vi "LCR_Logfile.vi"(4 "Data cluster":T1, 6 "Time Stamp":timestamp format="%<%x %.3X>T", 8 "error in":errorcluster, 9 "Data_In":T2 {"GUI Data Cluster"."SBR" format="%08b"}, 10 "Config_In":T4={"General"={"Config.ini"=path "", "Default Logging Path"=path ""}, "Hardware"={"Global T VAR"="", "Global B VAR"="", "VISAS"={"GEN COM"="", "SCOPE COM"="", "VNA COM"=""}}, "Operation"={"Operation Mode"=enum."Idle-Off", "Status"="", "NewLog?"=FALSE, "OvenWarn"=FALSE, "Scope Settings"={"TimeBase"=0.0, "VerticalScale"=4.0}}}) -> (0 "error out":errorcluster, 1 "Data_Out":T2 {"GUI Data Cluster"."SBR" format="%08b"}, 2 "Config_Out":T4={"General"={"Config.ini"=path "", "Default Logging Path"=path ""}, "Hardware"={"Global T VAR"="", "Global B VAR"="", "VISAS"={"GEN COM"="", "SCOPE COM"="", "VNA COM"=""}}, "Operation"={"Operation Mode"=enum."Idle-Off", "Status"="", "NewLog?"=FALSE, "OvenWarn"=FALSE, "Scope Settings"={"TimeBase"=0.0, "VerticalScale"=4.0}}}, 3 "File Failure":bool)   [LabVIEW 2021]
uses:
  Config_Cluster.ctl
  Mode_Enum.ctl
  Data_Cluster.ctl
  Measurement_Cluster.ctl
panel:
  in  "Status Ref":refnum<vi>
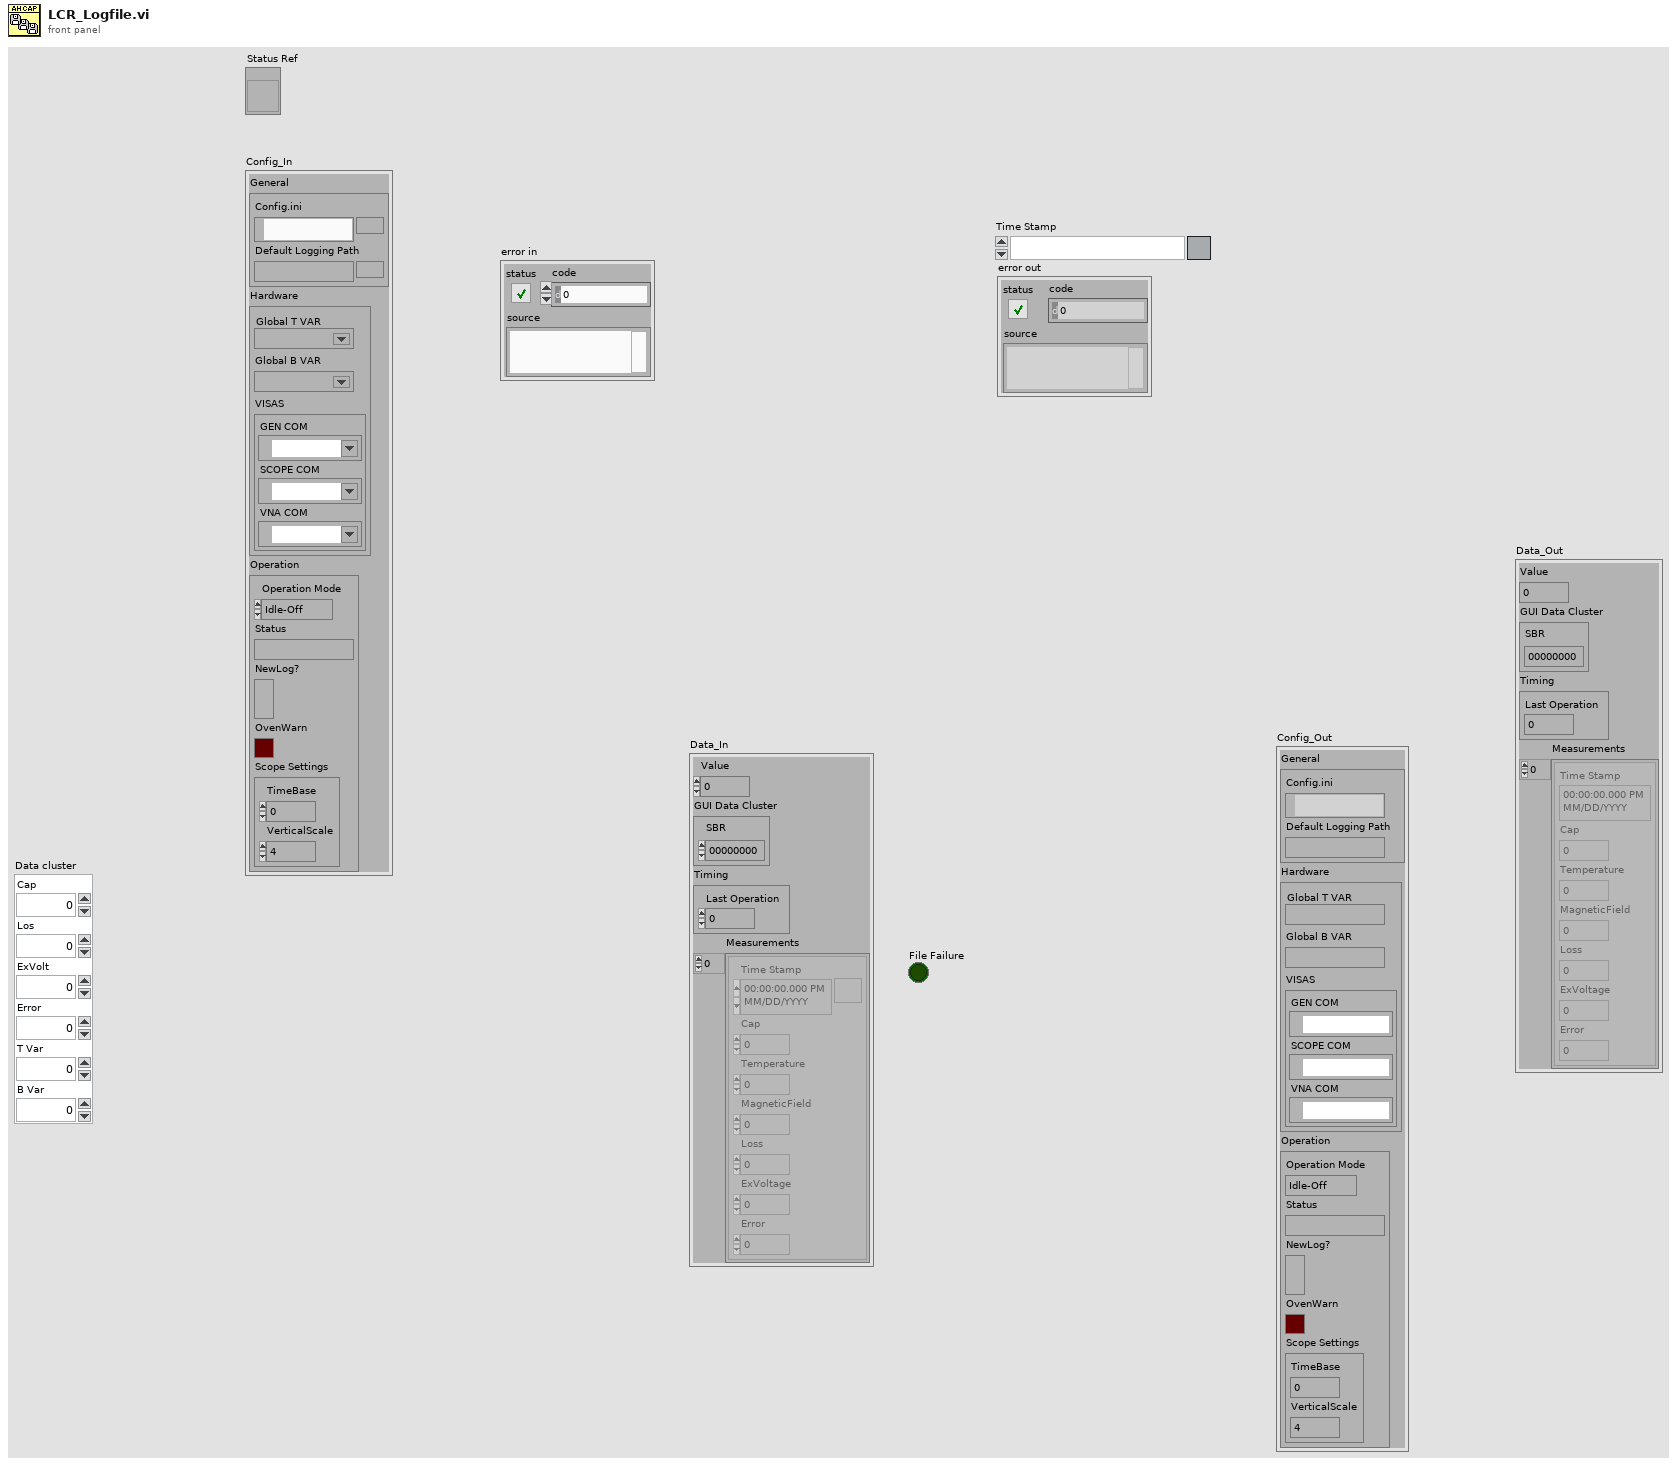
[diagram p1: front panel]
types:
  T1 = cluster{"Cap":dbl, "Los":dbl, "ExVolt":dbl, "Error":i32, "T Var":dbl, "B Var":dbl}
  T2 = typedef "Data_Cluster.ctl" = cluster{"Value":dbl, "GUI Data Cluster":cluster{"SBR":u16}, "Timing":cluster{"Last Operation":dbl}, "Measurements":T3[]}
  T3 = typedef "Measurement_Cluster.ctl" = cluster{"Time Stamp":timestamp, "Cap":dbl, "Temperature":dbl, "MagneticField":dbl, "Loss":dbl, "ExVoltage":dbl, "Error":dbl}
  T4 = typedef "Config_Cluster.ctl" = cluster{"General":cluster{"Config.ini":path, "Default Logging Path":path}, "Hardware":cluster{"Global T VAR":refnum<k21>, "Global B VAR":refnum<k21>, "VISAS":cluster{"GEN COM":refnum<visa-resource-name>, "SCOPE COM":refnum<visa-resource-name>, "VNA COM":refnum<visa-resource-name>}}, "Operation":cluster{"Operation Mode":T5, "Status":string, "NewLog?":bool, "OvenWarn":bool, "Scope Settings":cluster{"TimeBase":dbl, "VerticalScale":dbl}}}
  T5 = typedef "Mode_Enum.ctl" = enum16{"OvenNRDY", "Logging", "Idle-Off", "Idle"}
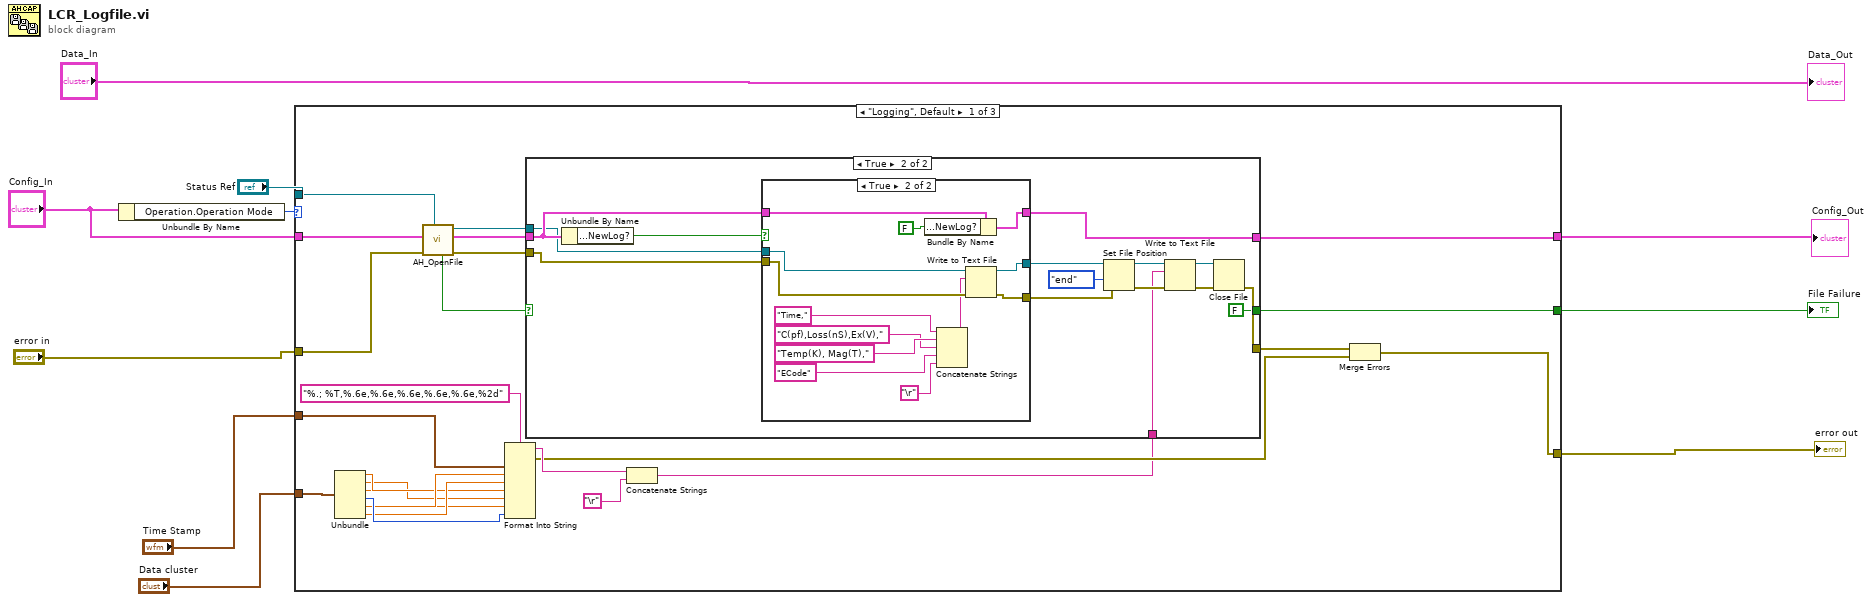
[diagram p0: block diagram]
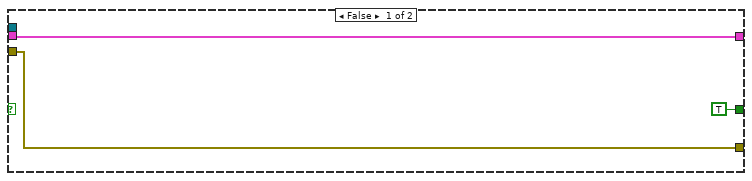
[diagram p2: hidden frame]
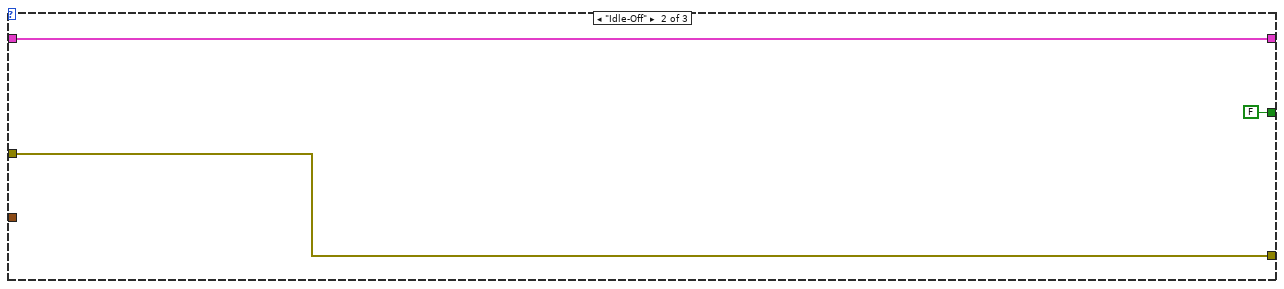
[diagram p4: hidden frame]
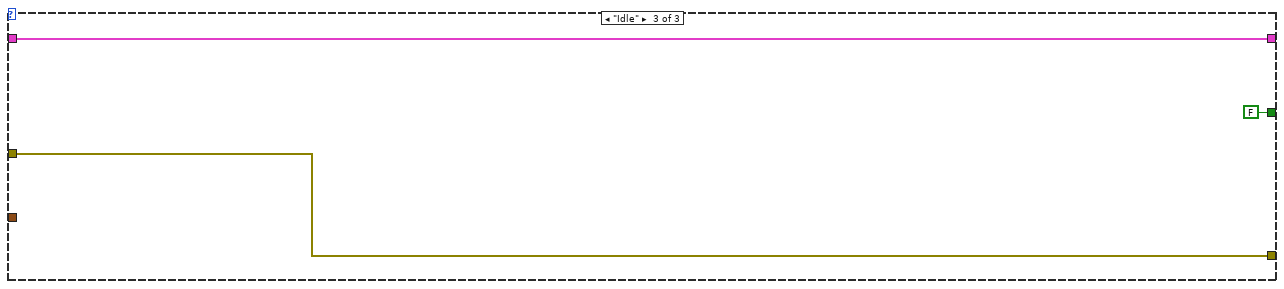
[diagram p5: hidden frame]
diagram:
  n1 = Unbundle By Name("Config_In") -> ("Operation.Operation Mode"=w6:T5)
  n2 = case shown="\"Logging\", Default" w6 {
    tunnel: "error in" -> [w27 w71 w74]
    tunnel: "Time Stamp" -> [w33 _ _]
    tunnel: [w19 w71 w74] -> w9
    tunnel: "Data cluster" -> [w32 _ _]
    tunnel: "Config_In" -> [w29 w70 w73]
    tunnel: "Status Ref" -> [w28 _ _]
    tunnel: [w18 w70 w73] -> w3
    tunnel: [w17 FALSE FALSE] -> w2
    frame "Logging", Default {
      n3 = Unbundle(w32) -> ("Cap"=w13:dbl, "Los"=w12:dbl, "ExVolt"=w11:dbl, "Error"=w16:i32, "T Var"=w15:dbl, "B Var"=w14:dbl)
      n4 = call "AH_OpenFile.vi"("Status Ref"=w28, "error in"=w27, "Config_Cluster"=w29) -> ("error out"=w23:errorcluster, "Config_Cluster Out"=w24:T4, "refnum out"=w25:refnum<file>, "FileOpen?"=w26:bool)  [unwired: 5 in]
      n5 = Format Into String(format string="%.; %T,%.6e,%.6e,%.6e,%.6e,%.6e,%2d", w33, w15, w14, w13, w12, w11, w16) -> (resulting string=w31:string, error out=w22:errorcluster)  [unwired: 2 in]
      n6 = Concatenate Strings(w31, "\r") -> (w21:string)
      n7 = case shown="True" w26 {
        tunnel: w25 -> [_ w42]
        tunnel: w24 -> [w36 w44]
        tunnel: w23 -> [w37 w41]
        tunnel: w21 -> [_ w46]
        tunnel: [w37 w45] -> w20
        tunnel: [w36 w43] -> w18
        tunnel: [TRUE FALSE] -> w17
        frame False {
        }
        frame True {
          n8 = Unbundle By Name(w44) -> ("Operation.NewLog?"=w52:bool)
          n9 = case shown="True" w52 {
            tunnel: w44 -> [w55 w68]
            tunnel: [w55 w67] -> w43
            tunnel: w42 -> [w54 w63]
            tunnel: w41 -> [w53 w62]
            tunnel: [w54 w65] -> w40
            tunnel: [w53 w64] -> w39
            frame False {
            }
            frame True {
              n10 = Bundle By Name(cluster=w68, "Operation.NewLog?"=FALSE) -> (w67:T4)
              n11 = Concatenate Strings("Time,", "Temp(K), Mag(T)," ("string"), "C(pf),Loss(nS),Ex(V),", "ECode" ("string"), "\r") -> (w60:string)
              n12 = Write to Text File(file (use dialog)=w63, text=w60, error in=w62) -> (refnum out=w65:refnum<file>, error out=w64:errorcluster)  [unwired: 1 in, 1 out]
            }
          }
          n13 = Set File Position(refnum=w40, from (0:start)=enum16{"start", "end", "current"}."end", error in=w39) -> (refnum out=w50:refnum<file>, error out=w51:errorcluster)  [unwired: 1 in]
          n14 = Write to Text File(file (use dialog)=w50, text=w46, error in=w51) -> (refnum out=w49:refnum<file>, error out=w48:errorcluster)  [unwired: 1 in, 1 out]
          n15 = Close File(refnum=w49, error in=w48) -> (error out=w45:errorcluster)  [unwired: 1 out]
        }
      }
      n16 = Merge Errors(w20, w22) -> (w19:errorcluster)
    }
    frame "Idle-Off" {
    }
    frame "Idle" {
    }
  }
  "error out" <- w9
  "Config_Out" <- w3
  "File Failure" <- w2
  "Data_Out" <- "Data_In"
